vi "Read_Position.vi"(6 "Error In":errorcluster, 8 "Node":u8, 9 "Serial In":refnum<visa-resource-name>) -> (0 "Error Out":errorcluster, 2 "Position":i32, 3 "Serial Out":refnum<visa-resource-name>)   [LabVIEW 2019]
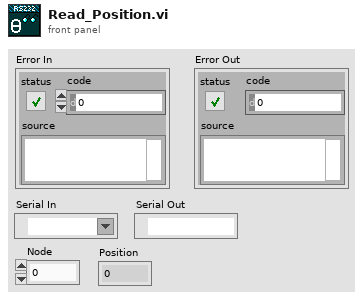
[diagram p1: front panel]
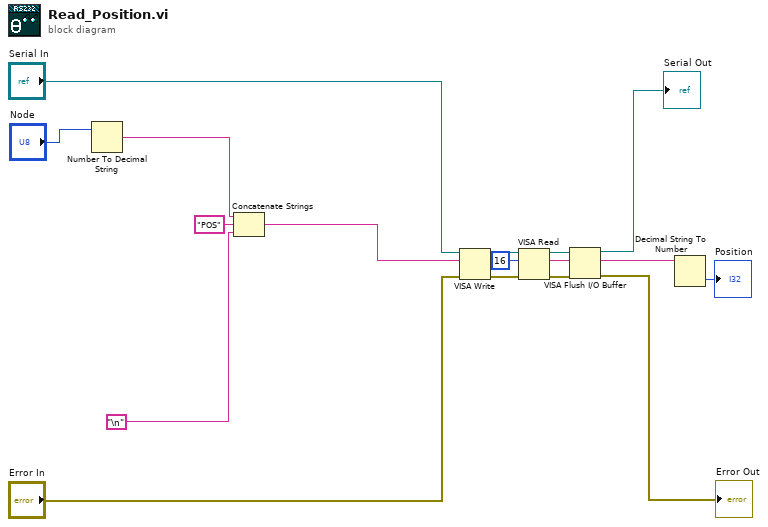
[diagram p0: block diagram]
diagram:
  n1 = Number To Decimal String(number="Node") -> (decimal integer string=w13:string)  [unwired: 1 in]
  n2 = Concatenate Strings(w13, "POS" ("string"), "\n") -> (w12:string)
  n3 = VISA Write(VISA resource name="Serial In", write buffer=w12, error in (no error)="Error In") -> (VISA resource name out=w9:refnum<visa-resource-name>, error out=w10:errorcluster)  [unwired: 1 out]
  n4 = VISA Read(VISA resource name=w9, byte count=u32 16, error in (no error)=w10) -> (VISA resource name out=w4:refnum<visa-resource-name>, read buffer=w7:string, error out=w5:errorcluster)  [unwired: 1 out]
  n5 = VISA Flush I/O Buffer(VISA resource name=w4, error in (no error)=w5) -> (VISA resource name out=→"Serial Out":refnum<visa-resource-name>, error out=→"Error Out":errorcluster)  [unwired: 1 in]
  n6 = Decimal String To Number(string=w7) -> (number=→"Position":i32)  [unwired: 2 in, 1 out]
